vi "Separated_Image.vi"(9 "Array":u32[][](array[numeric]), 10 "Array 2":u32[][](array[numeric])) -> (1 "path":path, 2 "stop 2":bool)   [LabVIEW 2016]
panel:
  in  "stop":bool
  out "Separated Channel":T1(plugin-control)
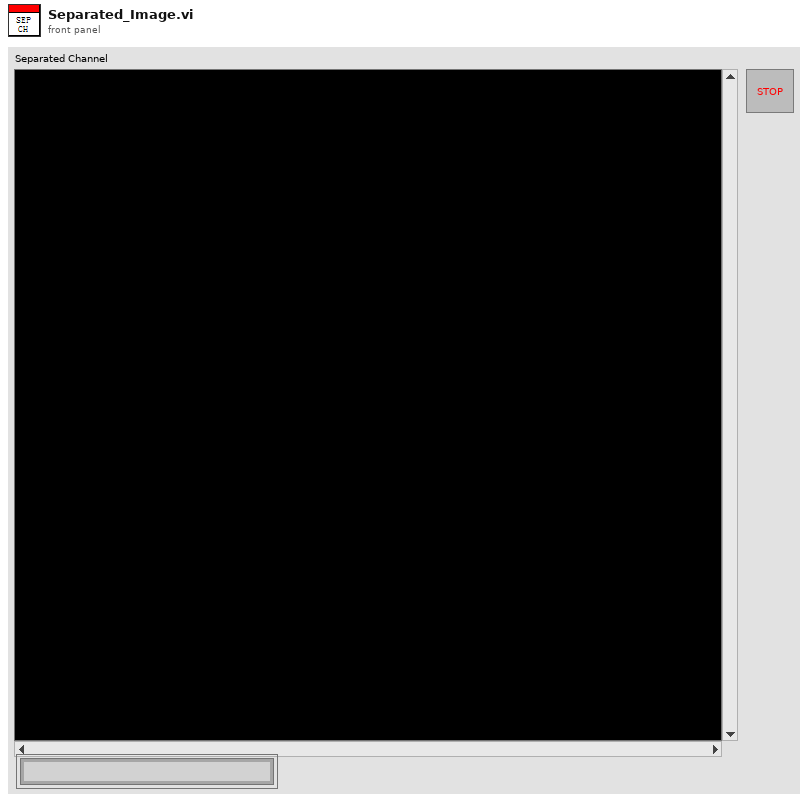
[diagram p1: front panel]
types:
  T1 = typedef "IMAQ Image.ctl" = refnum<image>
  T2 = typedef "Image Type" = u32
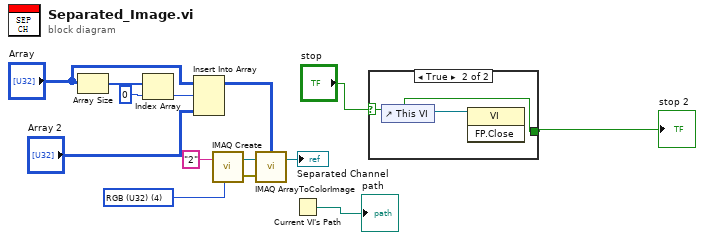
[diagram p0: block diagram]
diagram:
  w8 = T2 4 items=["Grayscale (U8)", "Grayscale (I16)", "Grayscale (SGL)", "Complex (CSG)", "RGB (U32)", "HSL (U32)", "RGB (U64)", "Grayscale (U16)"] ("Image Type")
  n1 = Array Size(array="Array") -> (size(s)=w12:i32[])
  n2 = Index Array(array=w12, index=0) -> (element=w10:i32)
  n3 = Insert Into Array(array="Array", index (row)=w10, new element="Array 2") -> (w5:u32[][])  [unwired: 1 in]
  n4 = call "IMAQ Create"("Image Name"="2", "Image Type"=w8) -> ("New Image"=w7:T1, "error out"=w6:errorcluster)  [unwired: 3 in]
  n5 = call "IMAQ ArrayToColorImage"("Image Pixels (U32)"=w5, "Image"=w7, "error in (no error)"=w6) -> ("Image Out"=→"Separated Channel":T1)  [unwired: 2 in, 1 out]
  n6 = Current VI's Path() -> (path=→"path":path)
  n7 = case shown="True" "stop" {
    selector: "stop" -> [w15 w16]
    tunnel: [w15 w16] -> w1
    frame False {
    }
    frame True {
      n8 = control-ref of="This VI"() -> (w17:refnum<vi>)
      n9 = invoke class="VI" method="FP.Close"(reference=w17) -> ()  [unwired: 2 in, 3 out]
    }
  }
  "stop 2" <- w1
